vi "Semver_string.vi"(8 "error in (no error)":errorcluster, 10 "Version":string) -> (0 "error out":errorcluster, 3 "Semver out":refnum<class "Semver.lvclass">)   [LabVIEW 2020, in "Semver.lvlib" / "Semver.lvclass"]
uses:
  Semver.lvclass
  Semver.lvclass/Semver.ctl
  <vilib>/Utility/error.llb/Error Cluster From Error Code.vi
  <vilib>/ErrorRing/Error Ring.xnode
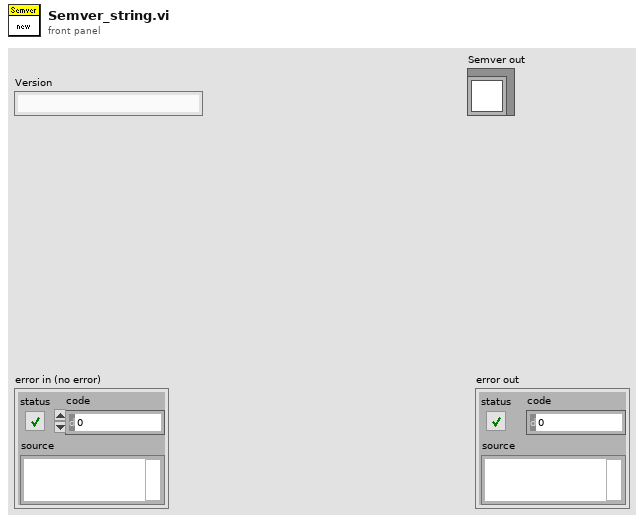
[diagram p1: front panel]
types:
  T1 = enum16{"Strip Chars", "Find Major", "Find Minor", "Find Patch", "Find Pre-Release", "Find Meta-Data"}
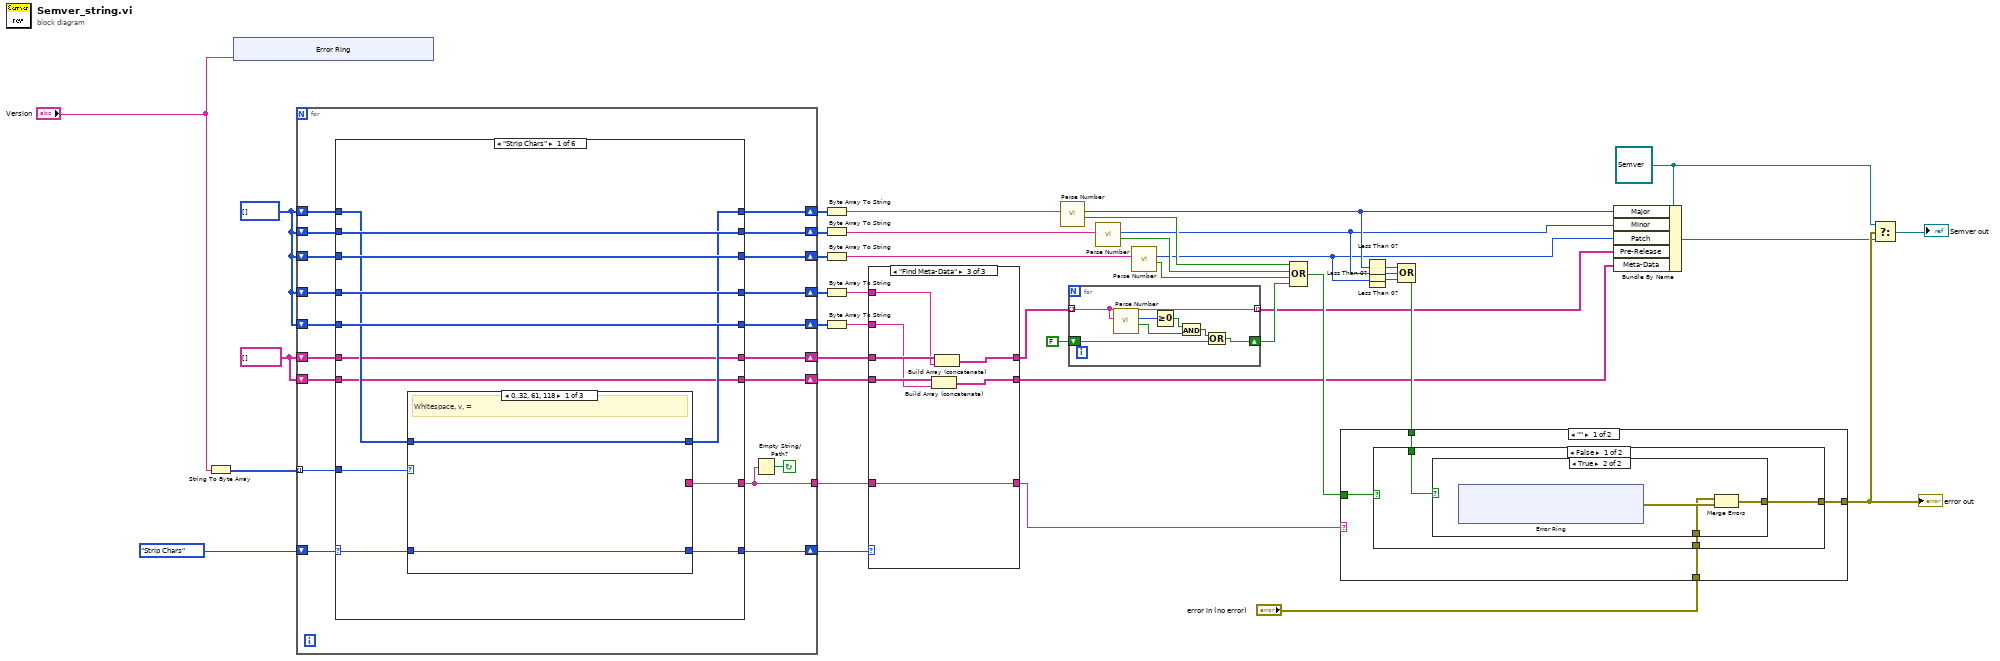
[diagram p0: block diagram]
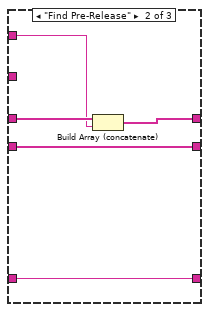
[diagram p3: hidden frame]
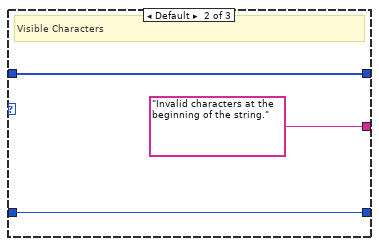
[diagram p4: hidden frame]
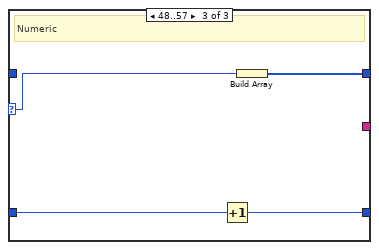
[diagram p5: hidden frame]
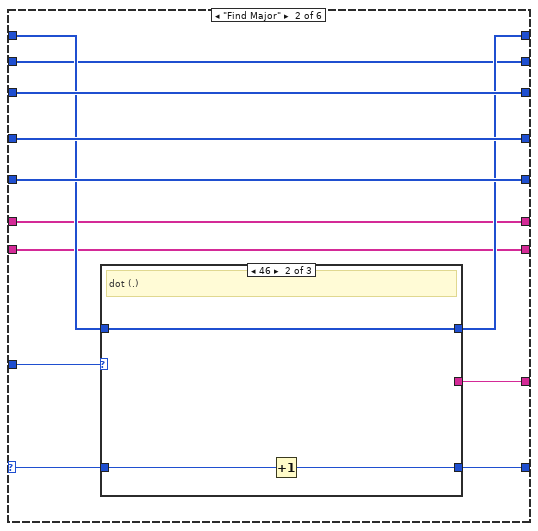
[diagram p6: hidden frame]
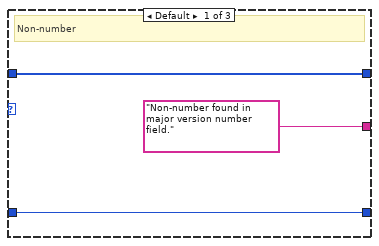
[diagram p7: hidden frame]
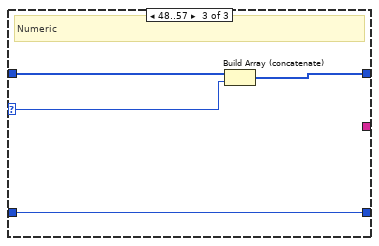
[diagram p8: hidden frame]
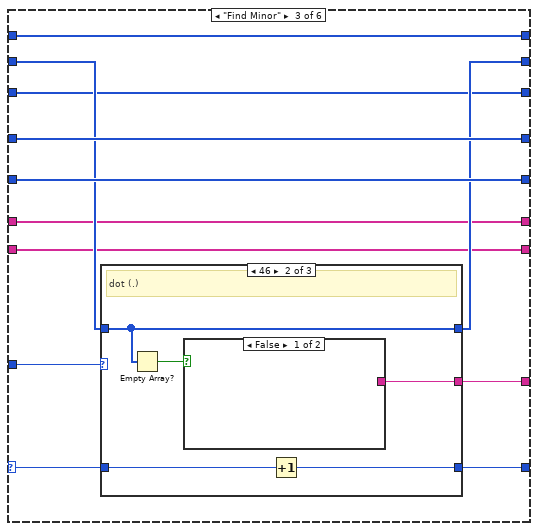
[diagram p9: hidden frame]
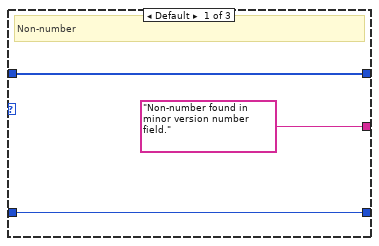
[diagram p10: hidden frame]
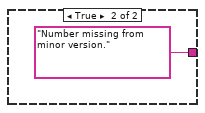
[diagram p11: hidden frame]
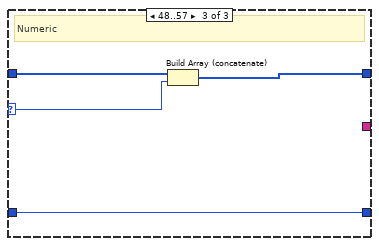
[diagram p12: hidden frame]
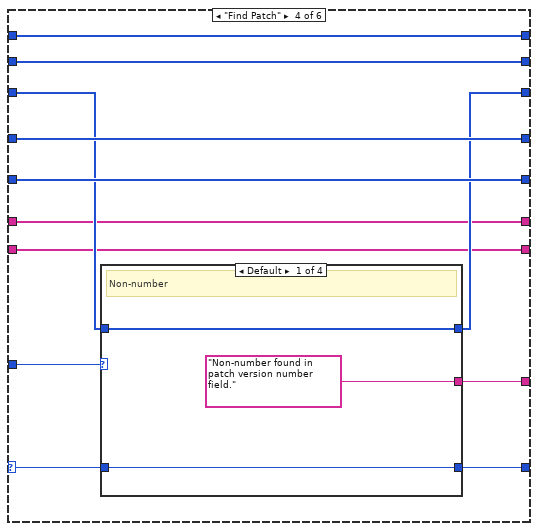
[diagram p13: hidden frame]
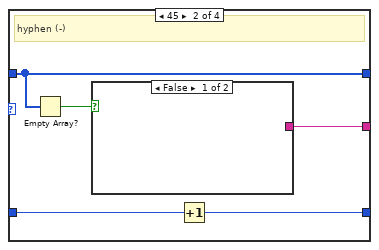
[diagram p14: hidden frame]
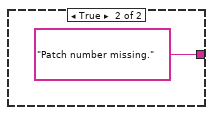
[diagram p15: hidden frame]
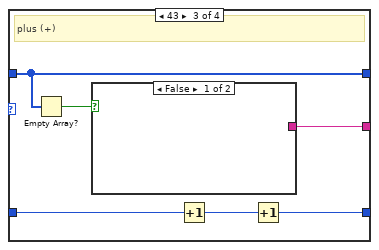
[diagram p16: hidden frame]
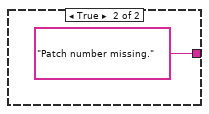
[diagram p17: hidden frame]
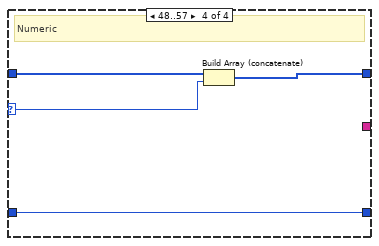
[diagram p18: hidden frame]
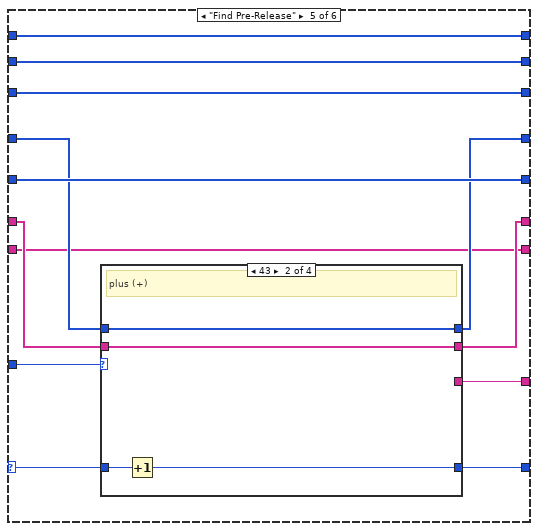
[diagram p19: hidden frame]
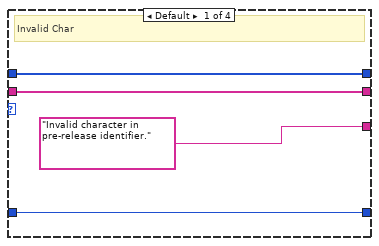
[diagram p20: hidden frame]
diagram:
  w1 = refnum<class "Semver.lvclass"> refnum ("Package Manager.lvlib:Semver.lvclass")
  w27 = string[] []
  w28 = u8[] []
  n1 = String To Byte Array(string="Version") -> (unsigned byte array=w29:u8[])
  n2 = xnode "Error Ring"("parameter 0"="Version") -> ()  [unwired: 1 out]
  n3 = for {
    tunnel: w29 -> [w48] mode=indexing
    shift-right: [w60] -> w26
    shift-left: w28 -> [w59]
    shift-right: [w58] -> w23
    shift-left: w28 -> [w57]
    shift-right: [w54] -> w22
    shift-left: w28 -> [w53]
    shift-right: [w55] -> w37
    shift-left: T1."Strip Chars" -> [w56]
    shift-right: [w52] -> w38
    shift-left: w28 -> [w51]
    shift-right: [w49] -> w39
    shift-left: w28 -> [w50]
    shift-right: [w47] -> w35
    shift-left: w27 -> [w46]
    shift-right: [w44] -> w34
    shift-left: w27 -> [w45]
    tunnel: [w43] -> w31
    stop <- w42 continue-if-true
    n4 = case shown="\"Strip Chars\"" w56 {
      selector: w56 -> [w67 w89 w112 w137 w172 w204]
      tunnel: [w64 w86 w110 w135 w170 w202] -> w60
      tunnel: w59 -> [w65 w87 w110 w135 w170 w202]
      tunnel: [w72 w82 w108 w134 w169 w201] -> w58
      tunnel: w57 -> [w72 w82 w109 w134 w169 w201]
      tunnel: [w66 w88 w111 w136 w171 w203] -> w55
      tunnel: [w71 w93 w104 w132 w168 w200] -> w54
      tunnel: w53 -> [w71 w93 w104 w133 w168 w200]
      tunnel: [w70 w92 w115 w140 w165 w196] -> w52
      tunnel: w51 -> [w70 w92 w115 w140 w166 w196]
      tunnel: [w69 w91 w114 w139 w167 w197] -> w49
      tunnel: w50 -> [w69 w91 w114 w139 w167 w198]
      tunnel: w48 -> [w68 w90 w113 w138 w173 w205]
      tunnel: [w63 w85 w107 w131 w163 w199] -> w47
      tunnel: w46 -> [w63 w85 w107 w131 w164 w199]
      tunnel: w45 -> [w62 w84 w106 w130 w162 w195]
      tunnel: [w62 w84 w106 w130 w162 w194] -> w44
      tunnel: [w61 w83 w105 w129 w161 w193] -> w43
      frame "Strip Chars" {
        n5 = case shown="0..32, 61, 118" w68 {
          selector: w68 -> [_ _ w79]
          tunnel: w67 -> [w74 w77 w81]
          tunnel: [w74 w77 w80] -> w66
          tunnel: w65 -> [w73 w76 _]
          tunnel: [w73 w76 w78] -> w64
          tunnel: [_ "Invalid characters at the beginning of the string." _] -> w61
          frame 0..32, 61, 118 {
            # "Whitespace, v, ="
          }
          frame Default {
            # "Visible Characters"
          }
          frame 48..57 {
            # "Numeric"
            n6 = Increment(x=w81) -> (x+1=w80:T1)
            n7 = Build Array(w79) -> (w78:u8[])
          }
        }
      }
      frame "Find Major" {
        n8 = case shown="46" w90 {
          selector: w90 -> [_ _ w100]
          tunnel: w89 -> [w96 w99 w103]
          tunnel: [w96 w97 w103] -> w88
          tunnel: w87 -> [w95 w98 w102]
          tunnel: [w95 w98 w101] -> w86
          tunnel: ["Non-number found in major version number field." _ _] -> w83
          frame Default {
            # "Non-number"
          }
          frame 46 {
            # "dot (.)"
            n9 = Increment(x=w99) -> (x+1=w97:T1)
          }
          frame 48..57 {
            # "Numeric"
            n10 = Build Array (concatenate)(w102, w100) -> (w101:u8[])
          }
        }
      }
      frame "Find Minor" {
        n11 = case shown="46" w113 {
          selector: w113 -> [_ _ w125]
          tunnel: w112 -> [w118 w123 w128]
          tunnel: [w118 w122 w128] -> w111
          tunnel: w109 -> [w117 w120 w127]
          tunnel: [w117 w120 w126] -> w108
          tunnel: ["Non-number found in minor version number field." w121 _] -> w105
          frame Default {
            # "Non-number"
          }
          frame 46 {
            # "dot (.)"
            n12 = Empty Array?(array=w120) -> (empty?=w119:bool)
            n13 = case shown="False" w119 {
              tunnel: [_ "Number missing from minor version."] -> w121
              frame False {
              }
              frame True {
              }
            }
            n14 = Increment(x=w123) -> (x+1=w122:T1)
          }
          frame 48..57 {
            # "Numeric"
            n15 = Build Array (concatenate)(w127, w125) -> (w126:u8[])
          }
        }
      }
      frame "Find Patch" {
        n16 = case shown="Default" w138 {
          selector: w138 -> [_ _ _ w157]
          tunnel: w137 -> [w143 w148 w155 w160]
          tunnel: [w143 w147 w153 w160] -> w136
          tunnel: w133 -> [w142 w145 w151 w159]
          tunnel: [w142 w145 w151 w158] -> w132
          tunnel: ["Non-number found in patch version number field." w146 w152 _] -> w129
          frame Default {
            # "Non-number"
          }
          frame 45 {
            # "hyphen (-)"
            n17 = Empty Array?(array=w145) -> (empty?=w144:bool)
            n18 = case shown="False" w144 {
              tunnel: [_ "Patch number missing."] -> w146
              frame False {
              }
              frame True {
              }
            }
            n19 = Increment(x=w148) -> (x+1=w147:T1)
          }
          frame 43 {
            # "plus (+)"
            n20 = Empty Array?(array=w151) -> (empty?=w150:bool)
            n21 = case shown="False" w150 {
              tunnel: [_ "Patch number missing."] -> w152
              frame False {
              }
              frame True {
              }
            }
            n22 = Increment(x=w155) -> (x+1=w154:T1)
            n23 = Increment(x=w154) -> (x+1=w153:T1)
          }
          frame 48..57 {
            # "Numeric"
            n24 = Build Array (concatenate)(w159, w157) -> (w158:u8[])
          }
        }
      }
      frame "Find Pre-Release" {
        n25 = case shown="43" w173 {
          selector: w173 -> [_ _ _ w189]
          tunnel: w172 -> [w177 w181 w183 w192]
          tunnel: [w177 w180 w183 w192] -> w171
          tunnel: w166 -> [w176 w179 w182 w191]
          tunnel: [w176 w179 u8[] [] w190] -> w165
          tunnel: w164 -> [w175 w178 w186 w188]
          tunnel: [w175 w178 w185 w188] -> w163
          tunnel: ["Invalid character in pre-release identifier." _ _ _] -> w161
          frame Default {
            # "Invalid Char"
          }
          frame 43 {
            # "plus (+)"
            n26 = Increment(x=w181) -> (x+1=w180:T1)
          }
          frame 46 {
            # "dot (.)"
            n27 = Byte Array To String(unsigned byte array=w182) -> (string=w184:string)
            n28 = Build Array (concatenate)(w186, w184) -> (w185:string[])
          }
          frame 48..57, 65..90, 97..122 {
            # "A-Za-z"
            n29 = Build Array (concatenate)(w191, w189) -> (w190:u8[])
          }
        }
      }
      frame "Find Meta-Data" {
        n30 = case shown="46" w205 {
          selector: w205 -> [_ _ w217 w221]
          tunnel: w204 -> [w209 w211 w220 w225]
          tunnel: [w209 w211 w220 w225] -> w203
          tunnel: w198 -> [w208 w210 w219 w222]
          tunnel: [w208 u8[] [] w218 w224] -> w197
          tunnel: w195 -> [w207 w214 w216 w223]
          tunnel: [w207 w213 w216 w223] -> w194
          tunnel: ["Invalid character in pre-release identifier." _ _ _] -> w193
          frame Default {
            # "Invalid Char"
          }
          frame 46 {
            # "dot (.)"
            n31 = Byte Array To String(unsigned byte array=w210) -> (string=w212:string)
            n32 = Build Array (concatenate)(w214, w212) -> (w213:string[])
          }
          frame 65..90, 97..122 {
            # "A-Za-z"
            n33 = Build Array (concatenate)(w219, w217) -> (w218:u8[])
          }
          frame 48..57 {
            # "A-Za-z"
            n34 = Build Array (concatenate)(w222, w221) -> (w224:u8[])
          }
        }
      }
    }
    n35 = Empty String/Path?(string/path=w43) -> (empty?=w42:bool)
  }
  n36 = Byte Array To String(unsigned byte array=w26) -> (string=w25:string)
  n37 = Byte Array To String(unsigned byte array=w23) -> (string=w24:string)
  n38 = Byte Array To String(unsigned byte array=w22) -> (string=w21:string)
  n39 = Byte Array To String(unsigned byte array=w38) -> (string=w36:string)
  n40 = Byte Array To String(unsigned byte array=w39) -> (string=w33:string)
  n41 = case shown="\"Find Meta-Data\"" w37 {
    tunnel: w36 -> [_ w230 w237]
    tunnel: [w228 w231 w238] -> w17
    tunnel: w35 -> [w228 w233 w240]
    tunnel: [w227 w232 w236] -> w5
    tunnel: w34 -> [w227 w232 w239]
    tunnel: w33 -> [_ _ w235]
    tunnel: [w226 w229 w234] -> w32
    tunnel: w31 -> [w226 w229 w234]
    frame Default {
    }
    frame "Find Pre-Release" {
      n42 = Build Array (concatenate)(w233, w230) -> (w231:string[])
    }
    frame "Find Meta-Data" {
      n43 = Build Array (concatenate)(w239, w235) -> (w236:string[])
      n44 = Build Array (concatenate)(w240, w237) -> (w238:string[])
    }
  }
  n45 = call "Parse Number.vi"("String"=w25) -> ("Leading Zero?"=w20:bool, "Number"=w9:i32)  [unwired: 9 in]
  n46 = for {
    tunnel: [w247] -> w6 mode=indexing
    tunnel: w17 -> [w247] mode=indexing
    shift-right: [w242] -> w15
    shift-left: FALSE -> [w243]
    n47 = call "Parse Number.vi"("String"=w247) -> ("Leading Zero?"=w244:bool, "Number"=w246:i32)  [unwired: 9 in]
    n48 = Greater Or Equal To 0?(x=w246) -> (x >= 0?=w245:bool)
    n49 = And(x=w245, y=w244) -> (x .and. y?=w241:bool)
    n50 = Or(x=w241, y=w243) -> (x .or. y?=w242:bool)
  }
  n51 = call "Parse Number.vi"("String"=w24) -> ("Leading Zero?"=w19:bool, "Number"=w8:i32)  [unwired: 9 in]
  n52 = call "Parse Number.vi"("String"=w21) -> ("Leading Zero?"=w18:bool, "Number"=w7:i32)  [unwired: 9 in]
  n53 = Compound Arithmetic op=OR(w20, w19, w18, w15) -> (w14:bool)
  n54 = Less Than 0?(x=w9) -> (x < 0?=w13:bool)
  n55 = Less Than 0?(x=w8) -> (x < 0?=w12:bool)
  n56 = Less Than 0?(x=w7) -> (x < 0?=w11:bool)
  n57 = Compound Arithmetic op=OR(w13, w12, w11) -> (w10:bool)
  n58 = case shown="\"\"" w32 {
    selector: w32 -> [_ w275]
    tunnel: [w249 w272] -> w4
    tunnel: "error in (no error)" -> [w250 w273]
    tunnel: w14 -> [w251 _]
    tunnel: w10 -> [w248 _]
    frame "" {
      n59 = case shown="False" w251 {
        tunnel: w250 -> [w254 w265]
        tunnel: [w253 w266] -> w249
        tunnel: w248 -> [w252 _]
        frame False {
          n60 = case shown="True" w252 {
            tunnel: w254 -> [w255 w257]
            tunnel: [w255 w256] -> w253
            frame False {
            }
            frame True {
              n61 = xnode "Error Ring"() -> ("error out"=w258:errorcluster)
              n62 = Merge Errors(w257, w258) -> (w256:errorcluster)
            }
          }
        }
        frame True {
          n63 = xnode "Error Ring"() -> ("error out"=w264:errorcluster)
          n64 = Merge Errors(w265, w264) -> (w266:errorcluster)
        }
      }
    }
    frame Default {
      n65 = xnode "Error Ring"("parameter 0"=w275) -> ("error out"=w274:errorcluster)
      n66 = Merge Errors(w273, w274) -> (w272:errorcluster)
    }
  }
  "error out" <- w4
  n67 = Bundle By Name(cluster=w1, "Major"=w9, "Minor"=w8, "Patch"=w7, "Pre-Release"=w6, "Meta-Data"=w5) -> (w3:refnum<class "Semver.lvclass">)
  n68 = Select(t=w1, s=w4, f=w3) -> (s? t:f=→"Semver out":refnum<class "Semver.lvclass">)
